vi "Microscope.GetConfiguration.vi"(8 "error in (no error)":errorcluster, 11 "Microscope":refnum<class "Microscope.lvclass">) -> (0 "error out":errorcluster, 2 "Configuration":T1={"XY Stage"="", "Camera"="", "image output folder"=path "", "filetype"="png"}, 3 "Microscope out":refnum<class "Microscope.lvclass">)   [LabVIEW 2013, in "Microscope.lvclass"]
doc: "---------------------------------------------------------------\nJKI State Machine Objects™\nhttp://jki.net/state-machine-objects/\nCopyright (C) 2005-2015, JKI <info@jki.net>\nALL RIGHTS RESERVEDJKI State Machine Objects (SMO) 1.0.0.5\nJKI - JKI\nCopyright (c) 2016, JKI"
uses:
  Microscope.lvclass
  Typedefs/Configuration--Cluster.ctl
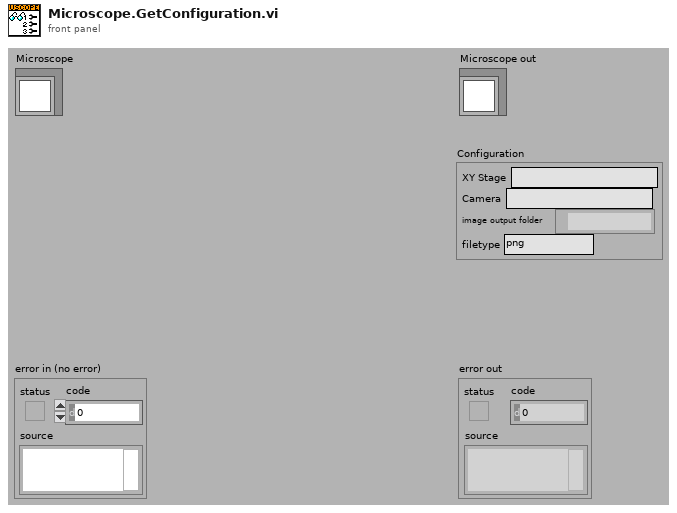
[diagram p1: front panel]
types:
  T1 = typedef "Microscope.lvclass/Configuration--Cluster.ctl" = cluster{"XY Stage":string, "Camera":string, "image output folder":path, "filetype":string}
  T2 = typedef "Microscope.lvclass/PrivateData--Ref.ctl" = refnum<data-value>
  T3 = typedef "Microscope.lvclass/PrivateData--Cluster.ctl" = cluster{"Public Events":T4, "Protected Events":T5, "Private Events":T6, "Dependencies":T7, "Configuration":T1}
  T4 = typedef "Microscope.lvclass/PublicEvents--Cluster.ctl" = cluster{"Value Changed":refnum<user-event>, "Initialized":refnum<user-event>}
  T5 = typedef "Microscope.lvclass/ProtectedEvents--Cluster.ctl" = cluster{"placeholder":refnum<user-event>}
  T6 = typedef "Microscope.lvclass/PrivateEvents--Cluster.ctl" = cluster{"New Value":refnum<user-event>, "Initialize":refnum<user-event>, "CaptureImageAtPosition":refnum<user-event>}
  T7 = typedef "Microscope.lvclass/Dependencies--Cluster.ctl" = cluster{"XYStage":refnum<class "XYStage.lvclass">, "Camera":refnum<class "Camera.lvclass">}
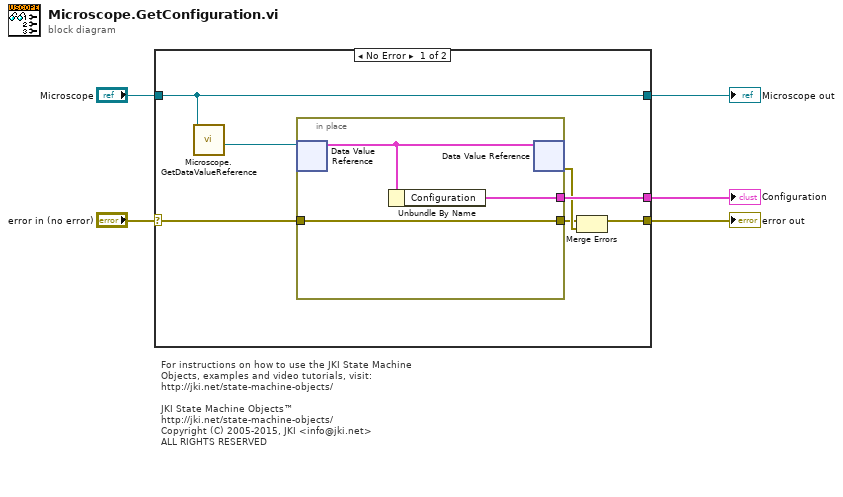
[diagram p0: block diagram]
diagram:
  # "For instructions on how to use the JKI State Machine Objects, examples and video tutorials, visit:\nhttp://jki.net/state-machine-objects/\n\nJKI State Machine Objects™\nhttp://jki.net/state-machine-objects/\nCopyright (C) 2005-2015, JKI <info@jki.net>\nALL RIGHTS RESERVED"
  n1 = case shown="No Error" "error in (no error)" {
    selector: "error in (no error)" -> [w12 w16]
    tunnel: "Microscope" -> [w7 w17]
    tunnel: [w10 w16] -> w5
    tunnel: [w7 w17] -> w4
    tunnel: [w11 _] -> w3
    frame No Error {
      n2 = call "Microscope.GetDataValueReference.vi"("Microscope"=w7) -> ("Ref"=w6:T2)  [unwired: 10 in]
      n3 = in-place {
        in-place-border: w12 -> [w15]
        in-place-border: [w15] -> w8
        in-place-border: [w14] -> w11
        n4 = in-place-dvr #1(w6) -> (w13:T3)  [unwired: 1 out]
        n5 = Unbundle By Name(w13) -> ("Configuration"=w14:T1)
        n6 = in-place-dvr #1(w13) -> (w9:errorcluster)  [unwired: 1 out]
      }
      n7 = Merge Errors(w8, w9) -> (w10:errorcluster)
    }
    frame Error {
      # "Upstream error or State Machine Object has not been created."
    }
  }
  "error out" <- w5
  "Microscope out" <- w4
  "Configuration" <- w3
